vi "LookupCommands.vi"(4 "CommandValues":string[](array[string]), 6 "CommandNames":string[](array[string]), 7 "Mode":enum16{"Read", "Initialize"}(ring), 10 "CommandName":string) -> (2 "CommandValue":string)   [LabVIEW 2010]
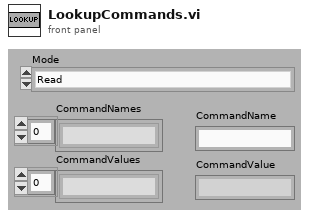
[diagram p1: front panel]
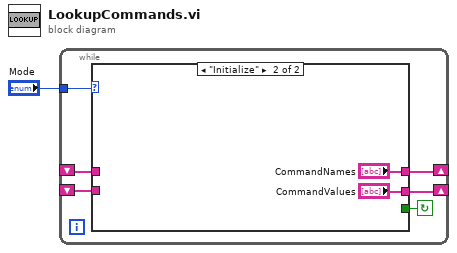
[diagram p0: block diagram]
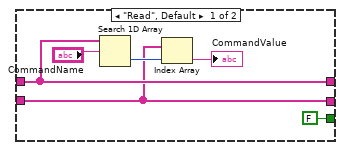
[diagram p2: hidden frame]
diagram:
  n1 = while {
    shift-right: [w5] -> _
    shift-left: _ -> [w3]
    tunnel: "Mode" -> [w7]
    shift-right: [w6] -> _
    shift-left: _ -> [w4]
    stop <- w2 continue-if-true
    n2 = case shown="\"Initialize\"" w7 {
      tunnel: [w11 "CommandNames"] -> w6
      tunnel: [w9 "CommandValues"] -> w5
      tunnel: w4 -> [w11 _]
      tunnel: w3 -> [w9 _]
      tunnel: [FALSE _] -> w2
      frame "Read", Default {
        n3 = Search 1D Array(1D array=w11, element="CommandName") -> (index of element=w10:i32)  [unwired: 1 in]
        n4 = Index Array(array=w9, index=w10) -> (element=→"CommandValue":string)
      }
      frame "Initialize" {
      }
    }
  }
